vi "Close IO.vi"(8 "error in (no error)":errorcluster, 11 "IO":T1) -> (0 "error out":errorcluster)   [LabVIEW 2021]
uses:
  IO_Type.ctl
  <vilib>/TSA/Event Log/Event_TextLog/Event_TextLog.lvclass
  Blackboard/Blackboard.lvclass
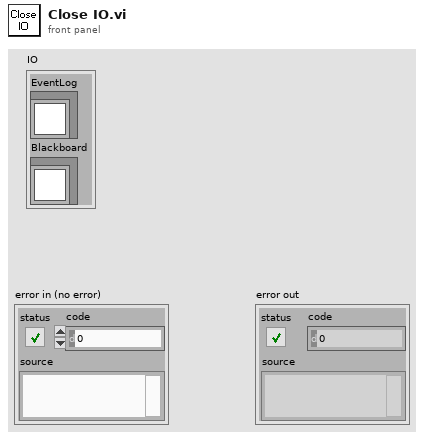
[diagram p1: front panel]
types:
  T1 = typedef "IO_Type.ctl" = cluster{"EventLog":refnum<class "Event_TextLog.lvclass">, "Blackboard":refnum<class "Blackboard.lvclass">}
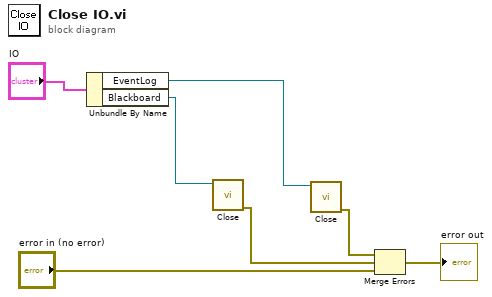
[diagram p0: block diagram]
diagram:
  n1 = Unbundle By Name("IO") -> ("EventLog"=w3:refnum<class "Event_TextLog.lvclass">, "Blackboard"=w2:refnum<class "Blackboard.lvclass">)
  n2 = call-dynamic "Close.vi"("bt_Blackboard in"=w2) -> ("error out"=w1:errorcluster)  [unwired: 9 in, 1 out]
  n3 = call-dynamic "Close.vi"("Event_TextLog in"=w3) -> ("error out"=w7:errorcluster)  [unwired: 9 in, 1 out]
  n4 = Merge Errors(w7, w1, "error in (no error)") -> (→"error out":errorcluster)
